vi "Point_Get_Attribute.vi"(8 "Error In":errorcluster, 9 "Attribute":string, 10 "Tag":string, 11 "Map":T1) -> (0 "Error Out":errorcluster, 1 "Value":string, 2 "Found?":bool, 3 "Map Out":T1)   [LabVIEW 2017, in "PointValueMap.lvlib"]
uses:
  <vilib>/addons/PointValueMap/PointValueMap.lvlib
  <vilib>/addons/PointValueMap/controls/PointMap.ctl
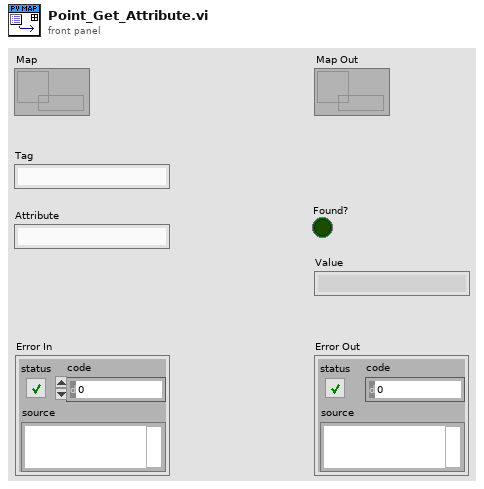
[diagram p1: front panel]
types:
  T1 = typedef "PointValueMap.lvlib/PointMap.ctl" = refnum<data-value>
  T2 = typedef "PointValueMap.lvlib/Point.ctl" = cluster{"Datatype":T3, "Timestamp":timestamp, "Value":variant, "Valid":bool}
  T3 = typedef "PointValueMap.lvlib/DataTypes.ctl" = enum16{"single", "double", "i32", "string", "variant"}
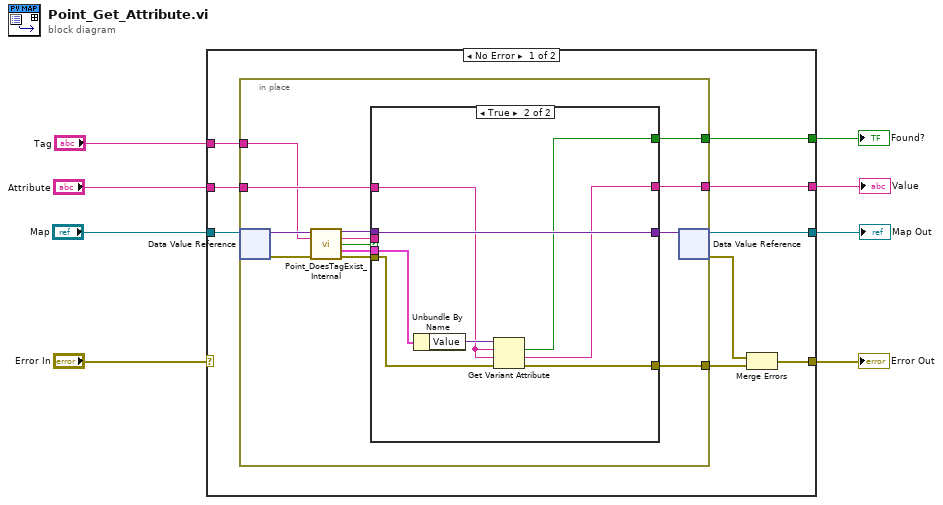
[diagram p0: block diagram]
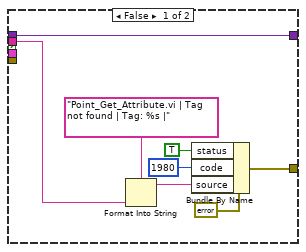
[diagram p2: hidden frame]
diagram:
  n1 = case shown="No Error" "Error In" {
    selector: "Error In" -> [_ w48]
    tunnel: "Map" -> [w17 w47]
    tunnel: "Tag" -> [w16 _]
    tunnel: [w13 w48] -> w7
    tunnel: "Attribute" -> [w12 _]
    tunnel: [w11 _] -> w4
    tunnel: [w10 w47] -> w1
    tunnel: [w9 _] -> w3
    frame No Error {
      n2 = in-place {
        in-place-border: w16 -> [w20]
        in-place-border: [w21] -> w14
        in-place-border: w12 -> [w30]
        in-place-border: [w22] -> w11
        in-place-border: [w23] -> w9
        n3 = in-place-dvr #1(w17) -> (w26:variant, w28:errorcluster)
        n4 = call <vilib>:"Point_DoesTagExist_Internal.vi"("Map"=w26, "Tag"=w20, "Error In"=w28) -> ("Map Out"=w25:variant, "Tag Out"=w19:string, "Tag Exists"=w24:bool, "Point"=w18:T2, "Error Out"=w27:errorcluster)  [unwired: 7 in, 1 out]
        n5 = case shown="True" w24 {
          tunnel: w30 -> [_ w43]
          tunnel: [_ w41] -> w22
          tunnel: [w32 w45] -> w29
          tunnel: [_ w42] -> w23
          tunnel: w27 -> [_ w40]
          tunnel: w25 -> [w32 w45]
          tunnel: [w33 w39] -> w21
          tunnel: w19 -> [w31 _]
          tunnel: w18 -> [_ w46]
          frame False {
            n6 = Format Into String(format string="Point_Get_Attribute.vi | Tag not found | Tag: %s |" ("source"), w31) -> (resulting string=w35:string)  [unwired: 2 in, 1 out]
            n7 = Bundle By Name(cluster=errorcluster {"status"=FALSE, "code"=0, "source"=""} ("Error Out"), "status"=TRUE, "code"=1980, "source"=w35) -> (w33:errorcluster)
          }
          frame True {
            n8 = Unbundle By Name(w46) -> ("Value"=w44:variant)
            n9 = Get Variant Attribute(Variant=w44, name=w43, default value (empty Variant)=w43, error in=w40) -> (found=w42:bool, value=w41:string, error out=w39:errorcluster)  [unwired: 1 out]
          }
        }
        n10 = in-place-dvr #1(w29) -> (w10:T1, w15:errorcluster)
      }
      n11 = Merge Errors(w15, w14) -> (w13:errorcluster)
    }
    frame Error {
    }
  }
  "Error Out" <- w7
  "Value" <- w4
  "Found?" <- w3
  "Map Out" <- w1
